vi "Finalize.vi"(8 "error in":errorcluster) -> (0 "error out":errorcluster, 2 "configuration string out":string)   [LabVIEW 2020, in "Ballard ARINC 429 Hardware Configuration.lvlib"]
uses:
  Ballard ARINC 429 Hardware Configuration.lvlib
  Constants.vi
panel:
  in  "configuration string":string
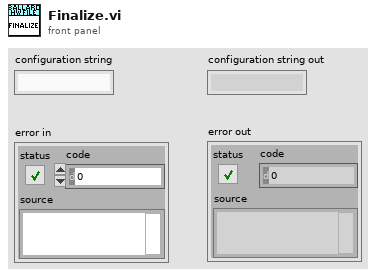
[diagram p1: front panel]
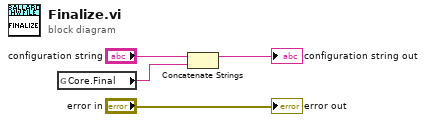
[diagram p0: block diagram]
diagram:
  n1 = global read "Constants.vi" "Core.Final"() -> (w3:string)
  n2 = Concatenate Strings("configuration string", w3) -> (→"configuration string out":string)
  "error out" <- "error in"
